vi "325 set Temp(SubVI).vi"(6 "Output (1:1)":u16(ring)=1 items=["1"=1, "2"=2], 7 "Input (0:A)":u16(ring)=1 items=["A", "B"], 8 "error in (no error)":errorcluster, 9 "Rate":dbl, 10 "Temperature":dbl=2.0, 11 "VISA Refnum in":refnum<visa-resource-name>="GPIB0::13::INSTR") -> (0 "error out":errorcluster, 3 "VISA resource name out":refnum<visa-resource-name>)   [LabVIEW 2019, in "SubVI.lvlib"]
uses:
  SubVI.lvlib
  lib/Lake Shore 325/Lake Shore 325.lvlib
panel:
  out "Sensor Data":dbl format="%.4f"
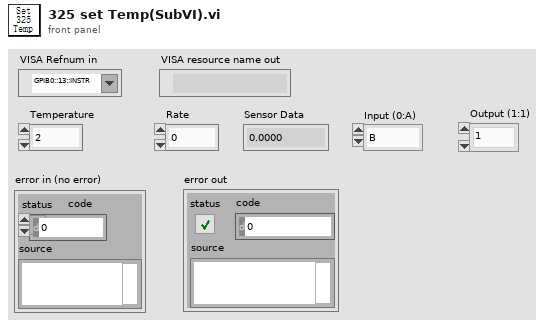
[diagram p1: front panel]
types:
  T1 = typedef "Semaphore RefNum" = refnum<k1>
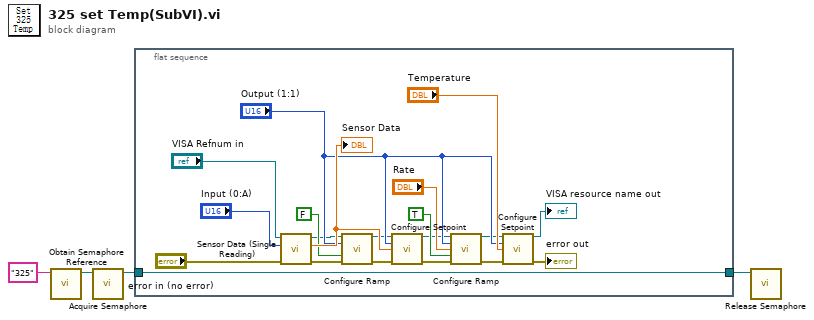
[diagram p0: block diagram]
diagram:
  n1 = call <vilib>:"Obtain Semaphore Reference.vi"("name (unnamed)"="325") -> ("semaphore"=w3:T1)  [unwired: 4 in, 2 out]
  n2 = call <vilib>:"Acquire Semaphore.vi"("semaphore"=w3) -> ("semaphore out"=w2:T1)  [unwired: 4 in, 2 out]
  n3 = flat-sequence {
    tunnel: w2 -> [w22]
    tunnel: [w22] -> w1
    frame #0 {
      n4 = call "Sensor Data (Single Reading).vi"("error in (no error)"="error in (no error)", "Sensor Input (0:A)"="Input (0:A)", "VISA resource name"="VISA Refnum in") -> ("error out"=w9:errorcluster, "Sensor Data"=w21:dbl, "VISA resource name out"=w14:refnum<visa-resource-name>)  [unwired: 6 in]
      "Sensor Data" <- w21
      n5 = call "Configure Ramp.vi"("VISA resource name"=w14, "Loop (1:Loop 1)"="Output (1:1)", "Setpoint Ramp (F: Off)"=FALSE ("Enable Setpoint Ramping (F: Off)"), "error in (no error)"=w9) -> ("VISA resource name out"=w13:refnum<visa-resource-name>, "error out"=w8:errorcluster)  [unwired: 10 in]
      n6 = call "Configure Setpoint.vi"("VISA resource name"=w13, "Loop (1:Loop 1)"="Output (1:1)", "Setpoint Value (0.0000)"=w21, "error in (no error)"=w8) -> ("VISA resource name out"=w12:refnum<visa-resource-name>, "error out"=w7:errorcluster)  [unwired: 10 in]
      n7 = call "Configure Ramp.vi"("VISA resource name"=w12, "Loop (1:Loop 1)"="Output (1:1)", "Rate Value (0.0)"="Rate", "Setpoint Ramp (F: Off)"=TRUE ("Enable Setpoint Ramping (F: Off)"), "error in (no error)"=w7) -> ("VISA resource name out"=w11:refnum<visa-resource-name>, "error out"=w6:errorcluster)  [unwired: 9 in]
      n8 = call "Configure Setpoint.vi"("VISA resource name"=w11, "Loop (1:Loop 1)"="Output (1:1)", "Setpoint Value (0.0000)"="Temperature", "error in (no error)"=w6) -> ("VISA resource name out"=→"VISA resource name out":refnum<visa-resource-name>, "error out"=→"error out":errorcluster)  [unwired: 10 in]
    }
  }
  n9 = call <vilib>:"Release Semaphore.vi"("semaphore"=w1) -> ()  [unwired: 5 in, 2 out]
